vi "Query Voltage.vi"(7 "Voltage Param (amplitude)":T1, 8 "error in (no error)":errorcluster, 10 "Channel (0: Channel 1)":T2 items=["Channel 1", "Channel 2"], 11 "VISA resource name":refnum<visa-resource-name>) -> (0 "error out":errorcluster, 1 "voltage":dbl[unit], 3 "VISA resource name out":refnum<visa-resource-name>)   [LabVIEW 2023, in "Tektronix AFG 3000 Series.lvlib"]
doc: "Queries the voltage of a Tektronix AFG 3000 series function generator; includes high, low, offset, or amplitude, as well as high and low voltage limits. <B>Note:</B> depending on which voltage you're querying and what the voltage units are set for (default: VPP), the return can be volts peak to peak, volts RMS, or even DBM."
uses:
  Tektronix AFG 3000 Series.lvlib
  controls.llb/Channel.ctl
  controls.llb/Voltage.ctl
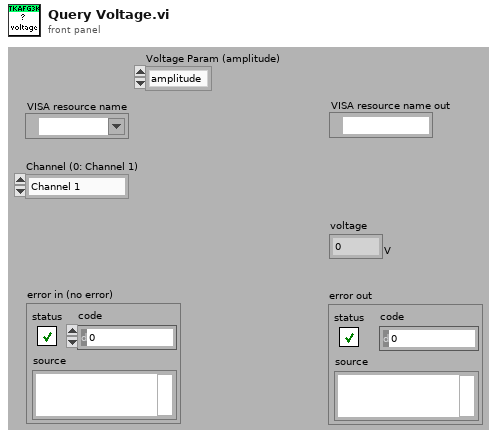
[diagram p1: front panel]
types:
  T1 = typedef "Voltage.ctl" = enum16{"amplitude", "offset", "high", "low", "high limit", "low limit"}
  T2 = typedef "Channel.ctl" = u16
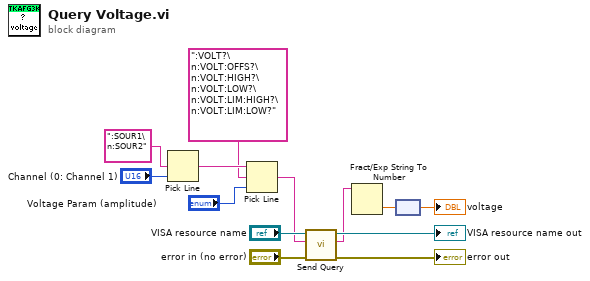
[diagram p0: block diagram]
diagram:
  n1 = Pick Line(multi-line string=":SOUR1\n:SOUR2", line index="Channel (0: Channel 1)") -> (output string=w4:string)  [unwired: 1 out]
  n2 = Pick Line(string ("")=w4, multi-line string=":VOLT?\n:VOLT:OFFS?\n:VOLT:HIGH?\n:VOLT:LOW?\n:VOLT:LIM:HIGH?\n:VOLT:LIM:LOW?", line index="Voltage Param (amplitude)") -> (output string=w2:string)
  n3 = call "Send Query.vi"("error in (no error)"="error in (no error)", "write buffer"=w2, "VISA resource name"="VISA resource name") -> ("error out"=→"error out":errorcluster, "read buffer"=w7:string, "VISA resource name out"=→"VISA resource name out":refnum<visa-resource-name>)  [unwired: 1 in, 5 out]
  n4 = Fract/Exp String To Number(string=w7) -> (number=w6:dbl)  [unwired: 4 out]
  n5 = node(w6) -> (→"voltage":dbl[unit])
